vi "Construct Connection Reference.vi"(11 "Connection":refnum<class "IConnection.lvclass">) -> (0 "error out":errorcluster, 3 "Connection Reference":refnum<data-value>)   [LabVIEW 2019, in "Connection Reference.lvlib" / "Connection Reference.lvclass"]
uses:
  <vilib>/gpm_packages/@cs/Network-interface/Source/Connection Reference/Connection Reference/Connection Reference.lvclass
  <vilib>/gpm_packages/@cs/Network-interface/Source/Connection Reference/IConnection/IConnection.lvclass
  <vilib>/gpm_packages/@cs/Network-interface/Source/Connection Reference/Connection Reference/Connection Reference.lvclass/Connection Reference.ctl
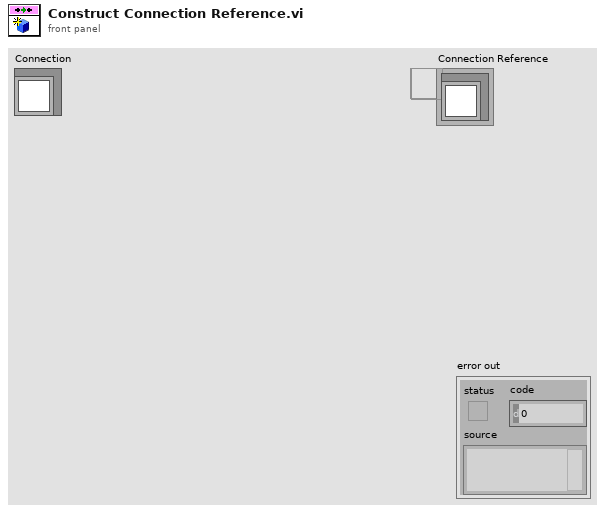
[diagram p1: front panel]
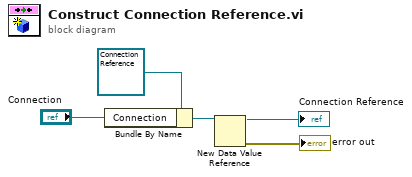
[diagram p0: block diagram]
diagram:
  n1 = Bundle By Name(cluster=refnum<class "Connection Reference.lvclass"> refnum ("Connection Reference in"), "Connection"="Connection") -> (w3:refnum<class "Connection Reference.lvclass">)
  n2 = New Data Value Reference(data value=w3) -> (data value reference=→"Connection Reference":refnum<data-value>, error out=→"error out":errorcluster)  [unwired: 1 in]
